vi "getSubArray3D.vi"(8 "error in (no error)":errorcluster, 9 "Index Array Cluster":T1, 10 "3D Array":dbl[][][](array[numeric]), 11 "MatOper in":refnum<class "MatOper.lvclass">) -> (0 "error out":errorcluster, 2 "Sub-Array":dbl[][][](array[numeric]), 3 "MatOper out":refnum<class "MatOper.lvclass">)   [LabVIEW 2016, in "OfcFunc.lvlib" / "MatOper.lvclass"]
doc: "Get the sub-array of the specific 3D array based on the index arrays."
uses:
  MatOper.lvclass
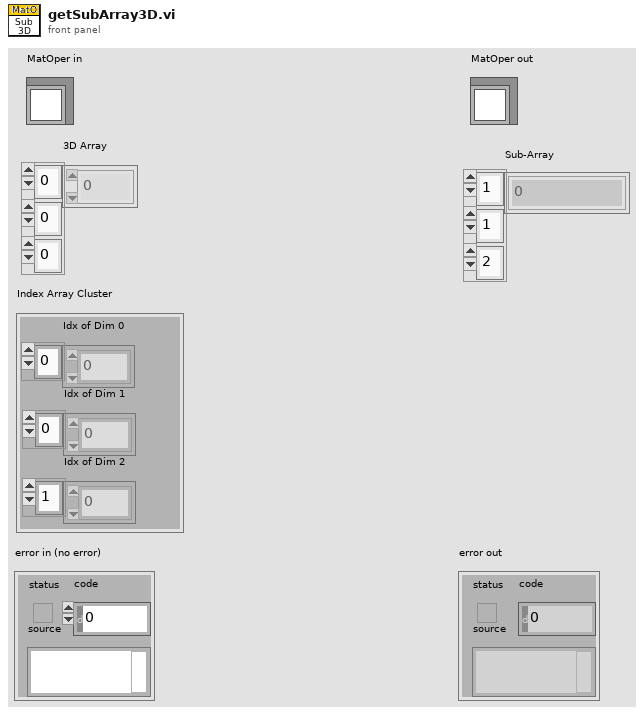
[diagram p1: front panel]
types:
  T1 = cluster{"Idx of Dim 0":i32[], "Idx of Dim 1":i32[], "Idx of Dim 2":i32[]}
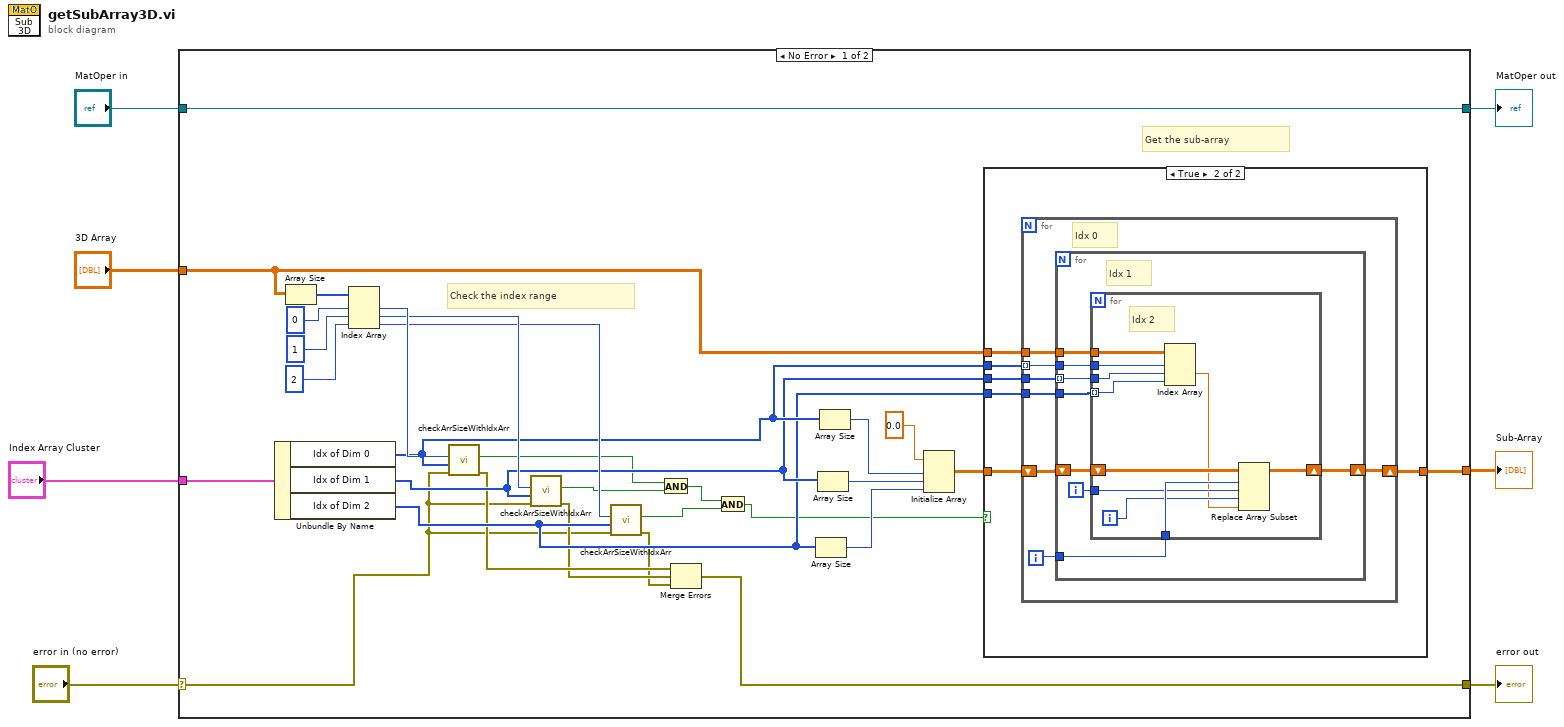
[diagram p0: block diagram]
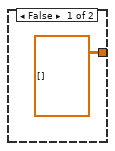
[diagram p2: hidden frame]
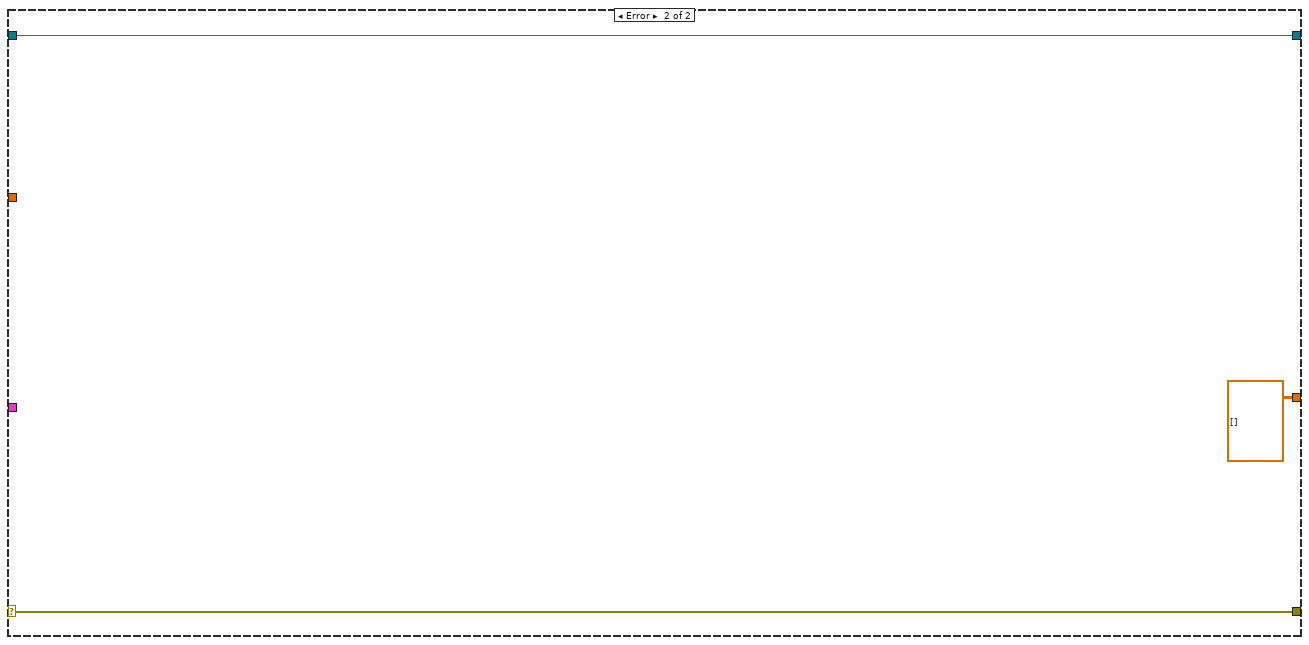
[diagram p3: hidden frame]
diagram:
  n1 = case shown="No Error" "error in (no error)" {
    selector: "error in (no error)" -> [w12 w71]
    tunnel: [w11 w71] -> w6
    tunnel: [w8 w70] -> w4
    tunnel: "MatOper in" -> [w8 w70]
    tunnel: [w13 dbl[][][] []] -> w3
    tunnel: "Index Array Cluster" -> [w10 _]
    tunnel: "3D Array" -> [w9 _]
    frame No Error {
      # "Check the index range"
      # "Get the sub-array"
      n2 = Unbundle By Name(w10) -> ("Idx of Dim 0"=w24:i32[], "Idx of Dim 1"=w23:i32[], "Idx of Dim 2"=w22:i32[])
      n3 = Array Size(array=w9) -> (size(s)=w31:i32[])
      n4 = Index Array(array=w31, index #1=0 ("index"), index #2=1 ("index"), index #3=2 ("index")) -> (element #1=w27:i32, element #2=w26:i32, element #3=w25:i32)
      n5 = call "checkArrSizeWithIdxArr.vi"("error in (no error)"=w12, "Idx Array"=w24, "Array Size"=w27) -> ("error out"=w16:errorcluster, "In Spec"=w21:bool)  [unwired: 6 in, 1 out]
      n6 = call "checkArrSizeWithIdxArr.vi"("error in (no error)"=w12, "Idx Array"=w23, "Array Size"=w26) -> ("error out"=w15:errorcluster, "In Spec"=w20:bool)  [unwired: 6 in, 1 out]
      n7 = call "checkArrSizeWithIdxArr.vi"("error in (no error)"=w12, "Idx Array"=w22, "Array Size"=w25) -> ("error out"=w14:errorcluster, "In Spec"=w19:bool)  [unwired: 6 in, 1 out]
      n8 = And(x=w21, y=w20) -> (x .and. y?=w18:bool)
      n9 = Merge Errors(w16, w15, w14) -> (w11:errorcluster)
      n10 = And(x=w18, y=w19) -> (x .and. y?=w17:bool)
      n11 = Array Size(array=w22) -> (size(s)=w34:i32)
      n12 = Array Size(array=w23) -> (size(s)=w32:i32)
      n13 = Array Size(array=w24) -> (size(s)=w33:i32)
      n14 = Initialize Array(0.0 ("element"), w33, w32, w34) -> (w35:dbl[][][])
      n15 = case shown="True" w17 {
        tunnel: w35 -> [_ w43]
        tunnel: [dbl[][][] [] w42] -> w13
        tunnel: w9 -> [_ w41]
        tunnel: w24 -> [_ w40]
        tunnel: w23 -> [_ w39]
        tunnel: w22 -> [_ w38]
        frame False {
        }
        frame True {
          n16 = for {
            tunnel: w41 -> [w50]
            shift-right: [w48] -> w42
            shift-left: w43 -> [w49]
            tunnel: w40 -> [w47] mode=indexing
            tunnel: w39 -> [w46]
            tunnel: w38 -> [w45]
            i -> [w44]
            # "Idx 0"
            n17 = for {
              tunnel: w50 -> [w58]
              shift-right: [w56] -> w48
              shift-left: w49 -> [w57]
              tunnel: w47 -> [w55]
              tunnel: w46 -> [w54] mode=indexing
              tunnel: w45 -> [w53]
              tunnel: w44 -> [w52]
              i -> [w51]
              # "Idx 1"
              n18 = for {
                tunnel: w58 -> [w68]
                shift-right: [w62] -> w56
                shift-left: w57 -> [w64]
                tunnel: w55 -> [w67]
                tunnel: w54 -> [w66]
                tunnel: w53 -> [w65] mode=indexing
                tunnel: w52 -> [w63]
                tunnel: w51 -> [w61]
                i -> [w60]
                # "Idx 2"
                n19 = Index Array(array=w68, index (dim 0)=w67, index (dim 1)=w66, index (dim 2)=w65) -> (element=w59:dbl)
                n20 = Replace Array Subset(array=w64, new element=w59, index (dim 0)=w63, index (dim 1)=w61, index (dim 2)=w60) -> (w62:dbl[][][])
              }
            }
          }
        }
      }
    }
    frame Error {
    }
  }
  "error out" <- w6
  "MatOper out" <- w4
  "Sub-Array" <- w3
